vi "TC_K_VtoC.vi"(11 "Thermocouple Voltage":dbl caption="热电偶电压" format="%0.6f") -> (3 "T(c)":dbl format="%#_16f")   [LabVIEW 2012]
doc: "功能：\n\nK型热电偶电压转换为摄氏度。\n\ncsxcs_366创建。"
uses:
  <vilib>/Analysis/polynomials.llb/Scalar Polynomial Evaluation (DBL).vi
  <vilib>/Analysis/NI_AALPro.lvlib
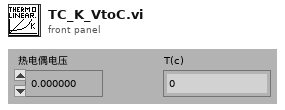
[diagram p1: front panel]
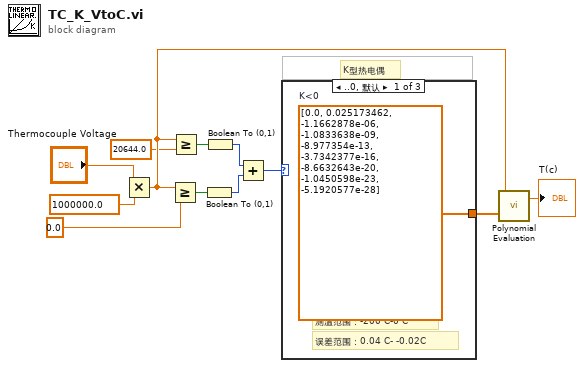
[diagram p0: block diagram]
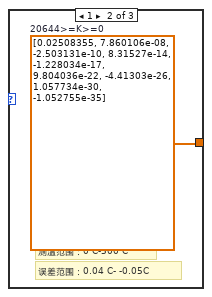
[diagram p2: hidden frame]
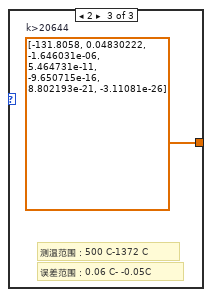
[diagram p3: hidden frame]
diagram:
  # "K型热电偶"
  n1 = Multiply(x="Thermocouple Voltage", y=1000000.0) -> (x*y=w8:dbl)
  n2 = Greater Or Equal?(x=w8, y=0.0) -> (x >= y?=w5:bool)
  n3 = Greater Or Equal?(x=w8, y=20644.0) -> (x >= y?=w6:bool)
  n4 = Boolean To (0,1)(Boolean=w5) -> (0, 1=w4:i16)
  n5 = Boolean To (0,1)(Boolean=w6) -> (0, 1=w3:i16)
  n6 = Add(x=w3, y=w4) -> (x+y=w2:i16)
  n7 = case shown="..0, 默认" w2 {
    tunnel: [w13 w14 w15] -> w1
    frame ..0, Default {
      w13 = dbl[] [0.0, 0.025173462, -1.1662878e-06, -1.0833638e-09, -8.977354e-13, -3.7342377e-16, -8.6632643e-20, -1.0450598e-23, -5.1920577e-28]  # K<0
      # "误差范围：0.04 C- -0.02C"
      # "测温范围：-200 C-0 C"
    }
    frame 1 {
      w14 = dbl[] [0.02508355, 7.860106e-08, -2.503131e-10, 8.31527e-14, -1.228034e-17, 9.804036e-22, -4.41303e-26, 1.057734e-30, -1.052755e-35]  # 20644>=K>=0
      # "误差范围：0.04 C- -0.05C"
      # "测温范围：0 C-500 C"
    }
    frame 2 {
      w15 = dbl[] [-131.8058, 0.04830222, -1.646031e-06, 5.464731e-11, -9.650715e-16, 8.802193e-21, -3.11081e-26]  # k>20644
      # "误差范围：0.06 C- -0.05C"
      # "测温范围：500 C-1372 C"
    }
  }
  n8 = call-poly <vilib>:"Polynomial Evaluation.vi"("P(x)"=w1, "a"=w8) -> ("P(a)"=→"T(c)":dbl)  [unwired: 1 out]
